vi "Read.vi"(8 "error in (no error)":errorcluster caption="entrée d'erreur (pas d'erreur)", 11 "Server TCP_IP P2110 en entrée":refnum<class "Server TCP_IP P2110.lvclass">) -> (0 "error out":errorcluster caption="sortie d'erreur", 3 "Server TCP_IP P2110 en sortie":refnum<class "Server TCP_IP P2110.lvclass">)   [LabVIEW 2020, in "Library Instrument & Equipement.lvlib" / "Library TCP IP.lvlib" / "Server TCP_IP P2110.lvclass"]
uses:
  Server TCP_IP P2110.lvclass
  C:/Users/ngarcin/OneDrive - Altyor/Standard TB/Class/TCP IP/Server TCP_IP (Default)/Server TCP_IP (Default).lvclass
  Server TCP_IP P2110.lvclass/Server TCP_IP P2110.ctl
  Commun VI/Library Commun.lvlib
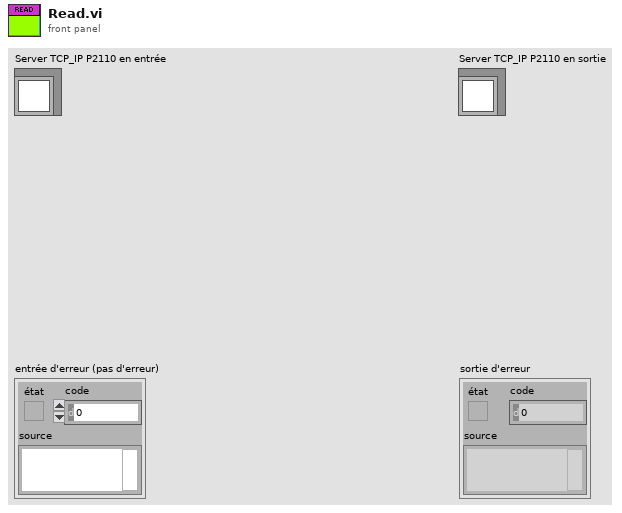
[diagram p1: front panel]
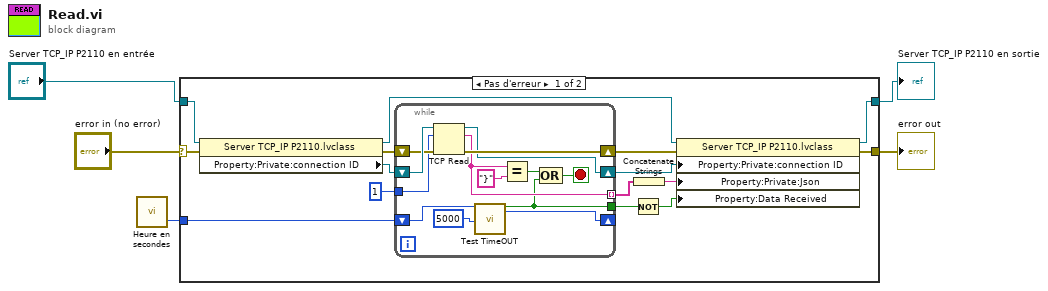
[diagram p0: block diagram]
diagram:
  n1 = call "Heure en secondes.vi"() -> ("Heure en milisecondes"=w1:u32)  [unwired: 2 in, 1 out]
  n2 = case shown="Pas d'erreur" "error in (no error)" {
    selector: "error in (no error)" -> [w14 w35]
    tunnel: [w13 w35] -> w2
    tunnel: [w15 w34] -> w3
    tunnel: "Server TCP_IP P2110 en entrée" -> [w16 w34]
    tunnel: w1 -> [w9 _]
    frame No Error {
      n3 = property class="Server TCP_IP P2110.lvclass"(reference=w16, error in=w14) -> (reference out=w17:refnum<class "Server TCP_IP P2110.lvclass">, error out=w19:errorcluster, "Property:Private:connection ID"=w20:refnum<k5>)
      n4 = while {
        tunnel: [w25] -> w12 mode=indexing
        tunnel: 1 ("octets à lire") -> [w29]
        shift-right: [w30] -> w11
        shift-left: w20 -> [w33]
        shift-right: [w31] -> w18
        shift-left: w19 -> [w32]
        shift-right: [w28] -> _
        shift-left: w9 -> [w27]
        tunnel: [w23] -> w8
        stop <- w22 stop-if-true
        n5 = TCP Read(connection ID=w33, bytes to read=w29, error in (no error)=w32) -> (connection ID out=w30:refnum<k5>, data out=w25:string, error out=w31:errorcluster)  [unwired: 2 in]
        n6 = call "Test TimeOUT.vi"("OLD Time"=w27, "TimeOut ms"=u32 5000) -> ("Timeout ?"=w23:bool, "NEW Time"=w28:u32)  [unwired: 13 in, 3 out]
        n7 = Equal?(x=w25, y="}") -> (x = y?=w21:bool)
        n8 = Compound Arithmetic op=OR ("Opérateur arithmétique")(w21, w23) -> (w22:bool)
      }
      n9 = Not(x=w8) -> (.not. x?=w7:bool)
      n10 = Concatenate Strings(w12) -> (w6:string)
      n11 = property class="Server TCP_IP P2110.lvclass"(reference=w17, error in=w18, "Property:Private:connection ID"=w11, "Property:Private:Json"=w6, "Property:Data Received"=w7) -> (reference out=w15:refnum<class "Server TCP_IP P2110.lvclass">, error out=w13:errorcluster)
    }
    frame Error {
    }
  }
  "error out" <- w2
  "Server TCP_IP P2110 en sortie" <- w3
